vi "Controls Log Monitor.vi"() -> ()   [LabVIEW 2013]
uses:
  <vilib>/Utility/miscctls.llb/LVDateTimeRec.ctl
  Controls Log Monitor.lvlib
  MTA Shift Toolbox.lvlib
panel:
  in  "Manual Report Shift Start Time":timestamp=timestamp(3497389200 s since 1904-01-01)
  in  "Failed Submission Sound File":path=path "\\\\beams-utility\\mta_archive$/mtarflv_shared/Shared/alertklaxon_clean.wav"
  out "Log Entry Text":string
  in  "Submit to ECL":bool=TRUE
  out "Last Entry ID":i32
  out "Reporting":bool
  in  "Report Now":bool
  in  "Log File Directory":path=path "C:/runs"
  in  "Successful Submission Sound File":path=path "\\\\beams-utility\\mta_archive$/mtarflv_shared/Shared/tng_torpedo_clean.wav"
  in  "stop":bool
  # "Controls Log Monitor.vi\nUpdated 7 March 2015\nby P. Lane"
  # "Coerced to the most recent fourth hour of the day."
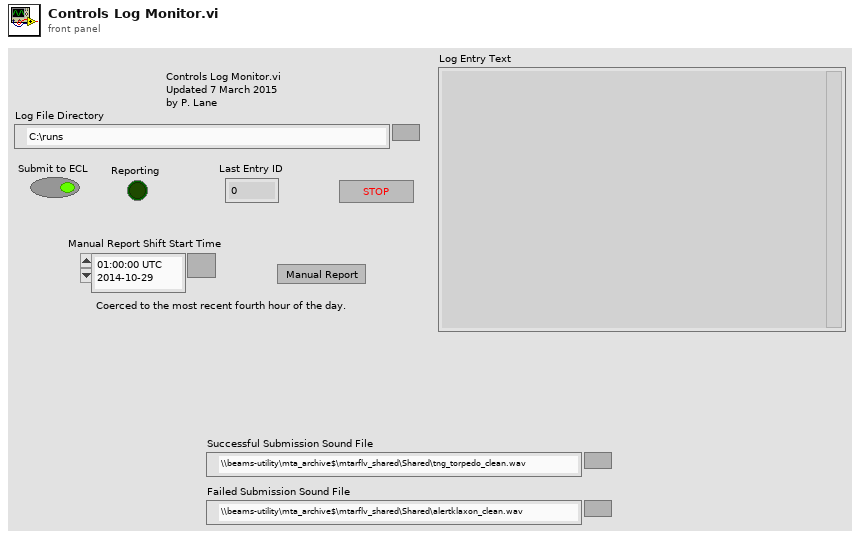
[diagram p1: front panel]
types:
  T1 = typedef "LVDateTimeRec.ctl" = cluster{"fractional second":dbl, "second":i32, "minute":i32, "hour":i32, "day of month":i32, "month":i32, "year":i32, "day of week":i32, "day of year":i32, "DST":i32}
  T2 = enum16{"Comissioning", "Comissioning/Detector", "Operations", "Operations/Absorber", "Operations/Beamline", "Operations/Controls", "Operations/Cryo", "Operations/DAQ", "Operations/Detectors", "Operations/Electrical", "Operations/Magnets", "Operations/Mechanical", "Operations/RF", "Operations/RF/201MHz", "Operations/RF/805MHz", "Operations/RF/PressurizedRF", "Operations/Safety", "Projects", "Projects/Logbook_Comments", "Projects/MTA_Operations", "Projects/MTA_Operations/Sandbox", "Sandbox", "Sandbox/Log", "Studies", "Studies/2010", "Studies/2010/2011_HPRF_test"}
  T3 = cluster{"Log File":path, "Pulse Number":u32, "Time Stamp":timestamp, "Event Type":enum16{"None", "Tune", "Periodic Capture", "Spark Trigger"}, "Probe Peak":dbl, "Probe/Reflected in Gate":dbl, "Gate Start Index":i32, "Gate End Index":i32, "Rise Tau":dbl, "Decay Tau":dbl, "Probe/Reflected after Gate":dbl, "Rise Slope":dbl, "Fall Slope":dbl, "Rise Duration":dbl, "Fall Duration":dbl, "Tuning Success":bool, "Signal Generator Frequency":dbl, "Signal Generator Amplitude":dbl, "Spark Trigger Name":string, "Spark Trigger Number":i32, "Reflected Max":dbl, "Reflected Max Index":i32, "Peak Index":i32}[]
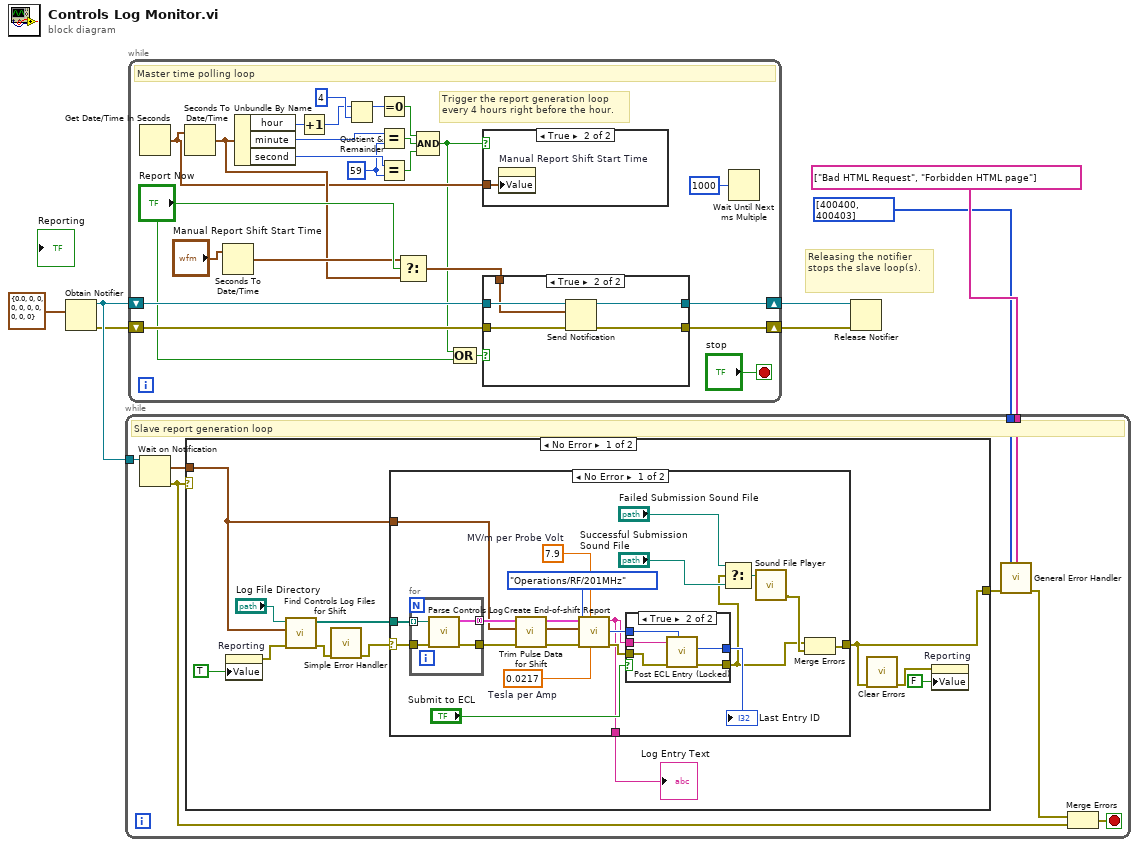
[diagram p0: block diagram]
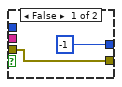
[diagram p2: hidden frame]
diagram:
  # "Releasing the notifier stops the slave loop(s)."
  n1 = Obtain Notifier(notification data type=T1 {"fractional second"=0.0, "second"=0, "minute"=0, "hour"=0, "day of month"=0, "month"=0, "year"=0, "day of week"=0, "day of year"=0, "DST"=0} ("date time rec")) -> (notifier out=w7:refnum<notifier>, error out=w6:errorcluster)  [unwired: 3 in, 1 out]
  n2 = while {
    tunnel: w7 -> [w15]
    tunnel: string[] ["Bad HTML Request", "Forbidden HTML page"] ("[user-defined descriptions]") -> [w13]
    tunnel: i32[] [400400, 400403] ("[user-defined codes]") -> [w12]
    stop <- w10 stop-if-true
    # "Slave report generation loop"
    n3 = Wait on Notification(notifier=w15) -> (notification=w14:T1, error out=w8:errorcluster)  [unwired: 1 in, 4 out]
    n4 = case shown="No Error" w8 {
      tunnel: w14 -> [w24 _]
      tunnel: [w16 _] -> w11
      frame No Error {
        n5 = property on="Reporting" class="Bool (strict)"("Value"=TRUE ("Reporting")) -> (error out=w21:errorcluster)  [unwired: 2 in, 1 out]
        n6 = call "Find Controls Log Files for Shift.vi"("error in (no error)"=w21, "Date/Time"=w24, "Log File Directory"="Log File Directory") -> ("error out"=w23:errorcluster, "Relevant Log Files"=w25:path[])  [unwired: 7 in]
        n7 = call <vilib>:"Simple Error Handler.vi"("error in (no error)"=w23) -> ("error out"=w22:errorcluster)  [unwired: 4 in, 4 out]
        n8 = case shown="No Error" w22 {
          selector: w22 -> [w34 w58]
          tunnel: w25 -> [w46 _]
          tunnel: w24 -> [w42 _]
          tunnel: [w33 w58] -> w16
          tunnel: [w36 _] -> w18
          frame No Error {
            w44 = 7.9  # MV/m per Probe Volt
            w35 = 0.0217  # Tesla per Amp
            n9 = for {
              tunnel: w46 -> [w57] mode=indexing
              tunnel: [w56] -> w45
              tunnel: [w55] -> w43 mode=concatenating
              tunnel: w34 -> [w54]
              n10 = call "Parse Controls Log.vi"("error in (no error)"=w54, "Controls Log File"=w57) -> ("error out"=w56:errorcluster, "Parsed Pulse Data"=w55:T3)  [unwired: 8 in]
            }
            n11 = call "Trim Pulse Data for Shift.vi"("date time rec"=w42, "Parsed Pulse Data"=w43) -> ("Shift Start Time"=w30:T1, "Shift Pulse Data"=w41:T3)  [unwired: 7 in, 1 out]
            n12 = call "Create End-of-shift Report.vi"("Tesla per Amp"=w35, "MV/m per Probe Volt"=w44, "error in (no error)"=w45, "date time rec"=w30, "Parsed Pulse Data"=w41) -> ("error out"=w39:errorcluster, "Log Entry Text"=w36:string)  [unwired: 5 in]
            n13 = case shown="True" "Submit to ECL" {
              tunnel: T2."Operations/RF/201MHz" ("Category") -> [_ w53]
              tunnel: w39 -> [w48 w52]
              tunnel: w36 -> [_ w51]
              tunnel: [w48 w50] -> w27
              tunnel: [-1 ("Entry ID") w49] -> w38
              frame False {
              }
              frame True {
                n14 = call "Post ECL Entry (Locked).vi"("Category"=w53, "error in (no error)"=w52, "Entry Text"=w51) -> ("error out"=w50:errorcluster, "Entry ID"=w49:i32)  [unwired: 7 in]
              }
            }
            "Last Entry ID" <- w38
            n15 = Select(t="Failed Submission Sound File", s=w27, f="Successful Submission Sound File") -> (s? t:f=w29:path)
            n16 = call "Sound File Player.vi"("Sound File Path"=w29) -> ("error out"=w28:errorcluster)  [unwired: 3 in, 1 out]
            n17 = Merge Errors(w27, w28) -> (w33:errorcluster)
          }
          frame Error {
          }
        }
        "Log Entry Text" <- w18
        n18 = call <vilib>:"Clear Errors.vi"("error in (no error)"=w16) -> ("error out"=w17:errorcluster)  [unwired: 6 in]
        n19 = property on="Reporting" class="Bool (strict)"(error in=w17, "Value"=FALSE ("Reporting")) -> ()  [unwired: 1 in, 2 out]
      }
      frame Error {
      }
    }
    n20 = call <vilib>:"General Error Handler.vi"("[user-defined codes]"=w12, "[user-defined descriptions]"=w13, "error in (no error)"=w11) -> ("error out"=w9:errorcluster)  [unwired: 8 in, 4 out]
    n21 = Merge Errors(w9, w8) -> (w10:errorcluster)
  }
  n22 = while {
    shift-right: [w80] -> w5
    shift-left: w6 -> [w79]
    shift-right: [w78] -> w4
    shift-left: w7 -> [w81]
    stop <- "stop" stop-if-true
    w60 = 59 ("y")
    # "Trigger the report generation loop\nevery 4 hours right before the hour."
    # "Master time polling loop"
    n23 = Get Date/Time In Seconds() -> (seconds since 1Jan1904=w69:timestamp)
    n24 = Seconds To Date/Time(time stamp (now)=w69) -> (date time rec=w70:T1)  [unwired: 1 in]
    n25 = Seconds To Date/Time(time stamp (now)="Manual Report Shift Start Time") -> (date time rec=w71:T1)  [unwired: 1 in]
    n26 = Unbundle By Name(w70) -> ("hour"=w67:i32, "minute"=w62:i32, "second"=w61:i32)
    n27 = Increment(x=w67) -> (x+1=w68:i32)
    n28 = Quotient & Remainder(x=w68, y=4) -> (x-y*floor(x/y)=w66:i32)  [unwired: 1 out]
    n29 = Equal To 0?(x=w66) -> (x = 0?=w64:bool)
    n30 = Equal?(x=w62, y=w60) -> (x = y?=w63:bool)
    n31 = Equal?(x=w61, y=w60) -> (x = y?=w59:bool)
    n32 = Select(t=w71, s="Report Now", f=w70) -> (s? t:f=w74:T1)
    n33 = Compound Arithmetic op=AND(w64, w63, w59) -> (w65:bool)
    n34 = Compound Arithmetic op=OR(w65, "Report Now") -> (w76:bool)
    n35 = case shown="True" w65 {
      tunnel: w69 -> [_ w83]
      frame False {
      }
      frame True {
        n36 = property on="Manual Report Shift Start Time" class="AbsTime (strict)"("Value"=w83) -> ()  [unwired: 2 in, 2 out]
      }
    }
    n37 = case shown="True" w76 {
      tunnel: w81 -> [w84 w90]
      tunnel: [w85 w89] -> w80
      tunnel: w79 -> [w85 w88]
      tunnel: [w84 w87] -> w78
      tunnel: w74 -> [_ w86]
      frame False {
      }
      frame True {
        n38 = Send Notification(notification=w86, notifier=w90, error in (no error)=w88) -> (notifier out=w87:refnum<notifier>, error out=w89:errorcluster)
      }
    }
    n39 = Wait Until Next ms Multiple(millisecond multiple=u32 1000 ("milliseconds to wait")) -> ()  [unwired: 1 out]
  }
  n40 = Release Notifier(notifier=w4, error in (no error)=w5) -> ()  [unwired: 4 out]
